vi "StopAModule.vi"(6 "ErrorArray In":errorcluster[](array[cluster]), 7 "Module Clone Reg":refnum<data-value>, 8 "error in (no error)":errorcluster, 10 "Module ID":i32, 11 "Module Name (e.g. Sensor, Digitizer, etc.)":string) -> (4 "ErrorArray Out":errorcluster[](array[cluster]))   [LabVIEW 2018, in "Test.lvclass"]
uses:
  Test.lvclass
  <userlib>/NIST/ModuleAdminLib/CloneRegistration/CloneRegistration.lvclass
  <userlib>/NIST/ModuleAdminLib/ModuleAdmin/ModuleAdmin.lvclass
  <userlib>/NIST/ModuleAdminLib/ModuleAdmin/ModuleAdmin.lvclass/ModuleAdmin.ctl
  <userlib>/NIST/ModuleAdminLib/ModuleAdmin/Accessors/Write CloneRegRef.vi
  <vilib>/Utility/error.llb/Error Cluster From Error Code.vi
  <vilib>/ErrorRing/Error Ring.xnode
  Sync/SyncModule/SyncModule.lvlib
  <userlib>/NIST/NISTErrorLib/NISTErrorLib.lvlib
  FGen/FgenShared/FgenShared.lvlib
  Digitizer/DigitizerShared/DigitizerShared.lvlib
  Scope/ScopeModule/ScopeModule.lvlib
  Sensor/SensorShared/SensorShared.lvlib
  Analysis/AnalysisModule/AnalysisModule.lvlib
  AcPwr/AcPwrModule/AcPwrModule.lvlib
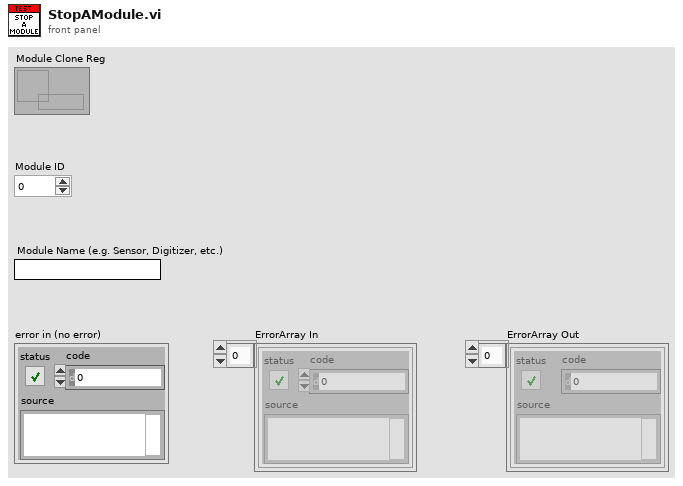
[diagram p1: front panel]
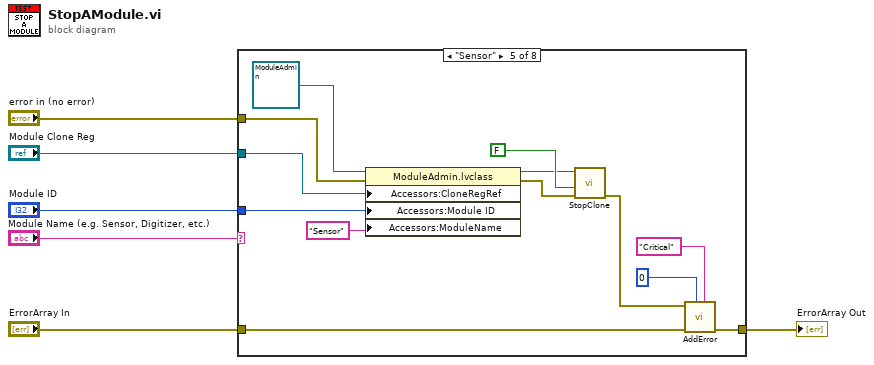
[diagram p0: block diagram]
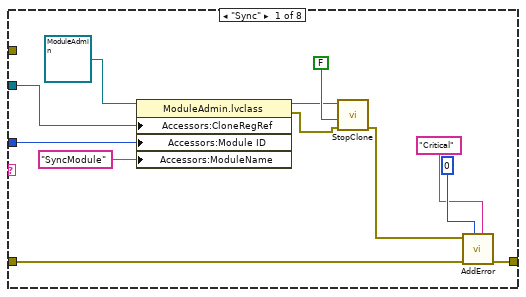
[diagram p2: hidden frame]
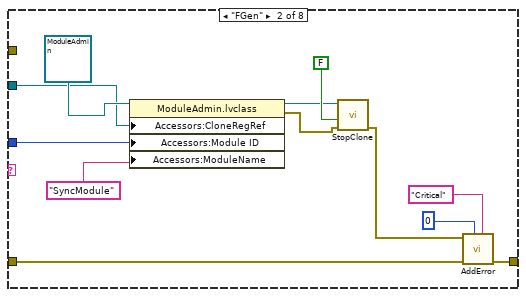
[diagram p3: hidden frame]
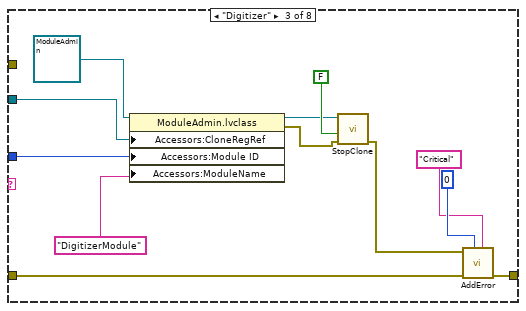
[diagram p4: hidden frame]
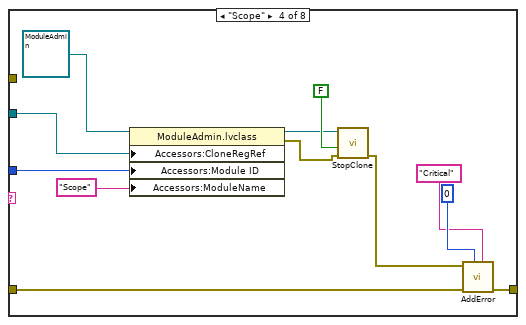
[diagram p5: hidden frame]
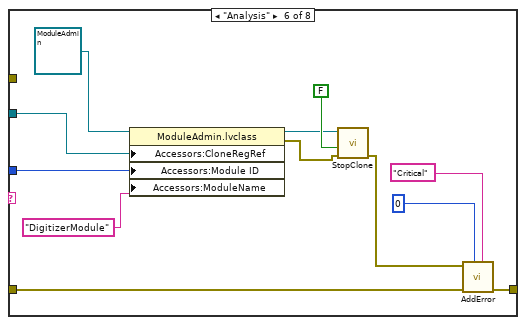
[diagram p6: hidden frame]
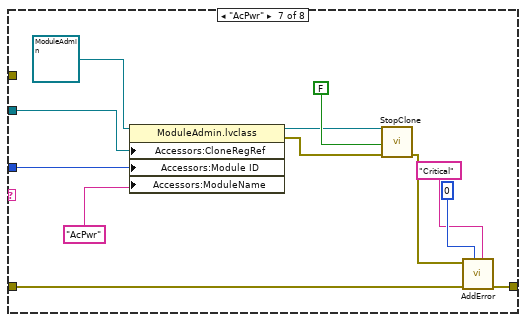
[diagram p7: hidden frame]
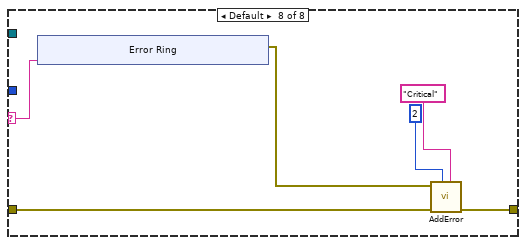
[diagram p8: hidden frame]
diagram:
  n1 = case shown="\"Sensor\"" "Module Name (e.g. Sensor, Digitizer, etc.)" {
    selector: "Module Name (e.g. Sensor, Digitizer, etc.)" -> [_ _ _ _ _ _ _ w97]
    tunnel: "ErrorArray In" -> [w8 w20 w32 w44 w57 w69 w84 w93]
    tunnel: [w12 w24 w36 w48 w61 w73 w87 w92] -> w3
    tunnel: "Module Clone Reg" -> [w17 w29 w41 w53 w66 w78 w90 _]
    tunnel: "Module ID" -> [w7 w19 w31 w43 w55 w68 w80 _]
    tunnel: "error in (no error)" -> [_ _ _ _ w56 _ _ _]
    frame "Sync" {
      n2 = property class="ModuleAdmin.lvclass"(reference=refnum<class "ModuleAdmin.lvclass"> refnum ("ModuleAdmin.lvlib:ModuleAdmin.lvclass"), "Accessors:CloneRegRef"=w17, "Accessors:Module ID"=w7, "Accessors:ModuleName"="SyncModule" ("ModuleName")) -> (reference out=w14:refnum<class "ModuleAdmin.lvclass">, error out=w13:errorcluster)  [unwired: 1 in]
      n3 = call "StopClone.vi"("error in (no error)"=w13, "Wait for Module to stop?"=FALSE, "ModuleAdmin"=w14) -> ("error out"=w9:errorcluster)  [unwired: 8 in]
      n4 = call <userlib>:"AddError.vi"("Severity"="Critical", "Priority"=u8 0, "ErrorArray In"=w8, "error in (no error)"=w9) -> ("ErrorArray Out"=w12:errorcluster[])  [unwired: 6 in, 1 out]
    }
    frame "FGen" {
      n5 = property class="ModuleAdmin.lvclass"(reference=refnum<class "ModuleAdmin.lvclass"> refnum ("ModuleAdmin.lvlib:ModuleAdmin.lvclass"), "Accessors:CloneRegRef"=w29, "Accessors:Module ID"=w19, "Accessors:ModuleName"="SyncModule" ("ModuleName")) -> (reference out=w26:refnum<class "ModuleAdmin.lvclass">, error out=w25:errorcluster)  [unwired: 1 in]
      n6 = call "StopClone.vi"("error in (no error)"=w25, "Wait for Module to stop?"=FALSE, "ModuleAdmin"=w26) -> ("error out"=w21:errorcluster)  [unwired: 8 in]
      n7 = call <userlib>:"AddError.vi"("Severity"="Critical", "Priority"=u8 0, "ErrorArray In"=w20, "error in (no error)"=w21) -> ("ErrorArray Out"=w24:errorcluster[])  [unwired: 6 in, 1 out]
    }
    frame "Digitizer" {
      n8 = property class="ModuleAdmin.lvclass"(reference=refnum<class "ModuleAdmin.lvclass"> refnum ("ModuleAdmin.lvlib:ModuleAdmin.lvclass"), "Accessors:CloneRegRef"=w41, "Accessors:Module ID"=w31, "Accessors:ModuleName"="DigitizerModule" ("ModuleName")) -> (reference out=w38:refnum<class "ModuleAdmin.lvclass">, error out=w37:errorcluster)  [unwired: 1 in]
      n9 = call "StopClone.vi"("error in (no error)"=w37, "Wait for Module to stop?"=FALSE, "ModuleAdmin"=w38) -> ("error out"=w33:errorcluster)  [unwired: 8 in]
      n10 = call <userlib>:"AddError.vi"("Severity"="Critical", "Priority"=u8 0, "ErrorArray In"=w32, "error in (no error)"=w33) -> ("ErrorArray Out"=w36:errorcluster[])  [unwired: 6 in, 1 out]
    }
    frame "Scope" {
      n11 = property class="ModuleAdmin.lvclass"(reference=refnum<class "ModuleAdmin.lvclass"> refnum ("ModuleAdmin.lvlib:ModuleAdmin.lvclass"), "Accessors:CloneRegRef"=w53, "Accessors:Module ID"=w43, "Accessors:ModuleName"="Scope" ("ModuleName")) -> (reference out=w50:refnum<class "ModuleAdmin.lvclass">, error out=w49:errorcluster)  [unwired: 1 in]
      n12 = call "StopClone.vi"("error in (no error)"=w49, "Wait for Module to stop?"=FALSE, "ModuleAdmin"=w50) -> ("error out"=w45:errorcluster)  [unwired: 8 in]
      n13 = call <userlib>:"AddError.vi"("Severity"="Critical", "Priority"=u8 0, "ErrorArray In"=w44, "error in (no error)"=w45) -> ("ErrorArray Out"=w48:errorcluster[])  [unwired: 6 in, 1 out]
    }
    frame "Sensor" {
      n14 = property class="ModuleAdmin.lvclass"(reference=refnum<class "ModuleAdmin.lvclass"> refnum ("ModuleAdmin.lvlib:ModuleAdmin.lvclass"), error in=w56, "Accessors:CloneRegRef"=w66, "Accessors:Module ID"=w55, "Accessors:ModuleName"="Sensor" ("ModuleName")) -> (reference out=w63:refnum<class "ModuleAdmin.lvclass">, error out=w62:errorcluster)
      n15 = call "StopClone.vi"("error in (no error)"=w62, "Wait for Module to stop?"=FALSE, "ModuleAdmin"=w63) -> ("error out"=w58:errorcluster)  [unwired: 8 in]
      n16 = call <userlib>:"AddError.vi"("Severity"="Critical", "Priority"=u8 0, "ErrorArray In"=w57, "error in (no error)"=w58) -> ("ErrorArray Out"=w61:errorcluster[])  [unwired: 6 in, 1 out]
    }
    frame "Analysis" {
      n17 = property class="ModuleAdmin.lvclass"(reference=refnum<class "ModuleAdmin.lvclass"> refnum ("ModuleAdmin.lvlib:ModuleAdmin.lvclass"), "Accessors:CloneRegRef"=w78, "Accessors:Module ID"=w68, "Accessors:ModuleName"="DigitizerModule" ("ModuleName")) -> (reference out=w75:refnum<class "ModuleAdmin.lvclass">, error out=w74:errorcluster)  [unwired: 1 in]
      n18 = call "StopClone.vi"("error in (no error)"=w74, "Wait for Module to stop?"=FALSE, "ModuleAdmin"=w75) -> ("error out"=w70:errorcluster)  [unwired: 8 in]
      n19 = call <userlib>:"AddError.vi"("Severity"="Critical", "Priority"=u8 0, "ErrorArray In"=w69, "error in (no error)"=w70) -> ("ErrorArray Out"=w73:errorcluster[])  [unwired: 6 in, 1 out]
    }
    frame "AcPwr" {
      n20 = property class="ModuleAdmin.lvclass"(reference=refnum<class "ModuleAdmin.lvclass"> refnum ("ModuleAdmin.lvlib:ModuleAdmin.lvclass"), "Accessors:CloneRegRef"=w90, "Accessors:Module ID"=w80, "Accessors:ModuleName"="AcPwr" ("ModuleName")) -> (reference out=w81:refnum<class "ModuleAdmin.lvclass">, error out=w88:errorcluster)  [unwired: 1 in]
      n21 = call "StopClone.vi"("error in (no error)"=w88, "Wait for Module to stop?"=FALSE, "ModuleAdmin"=w81) -> ("error out"=w83:errorcluster)  [unwired: 8 in]
      n22 = call <userlib>:"AddError.vi"("Severity"="Critical", "Priority"=u8 0, "ErrorArray In"=w84, "error in (no error)"=w83) -> ("ErrorArray Out"=w87:errorcluster[])  [unwired: 6 in, 1 out]
    }
    frame Default {
      n23 = xnode "Error Ring"("parameter 0"=w97) -> ("error out"=w94:errorcluster)
      n24 = call <userlib>:"AddError.vi"("Severity"="Critical", "Priority"=u8 2, "ErrorArray In"=w93, "error in (no error)"=w94) -> ("ErrorArray Out"=w92:errorcluster[])  [unwired: 6 in, 1 out]
    }
  }
  "ErrorArray Out" <- w3
